vi "Render Draw Line (Clusters).vi"(8 "error in":errorcluster, 9 "End":T1, 10 "Start":T1, 11 "Renderer Pointer":u32 format="%.0x") -> (0 "error out":errorcluster, 3 "Return":i32)   [LabVIEW 2015, in "LibSDL2.lvlib"]
uses:
  LibSDL2.lvlib
  SDL2 Utility/Point (I32).ctl
  DLL/SDL2.dll
  SDL2 Utility/SDL2 Utility.lvlib
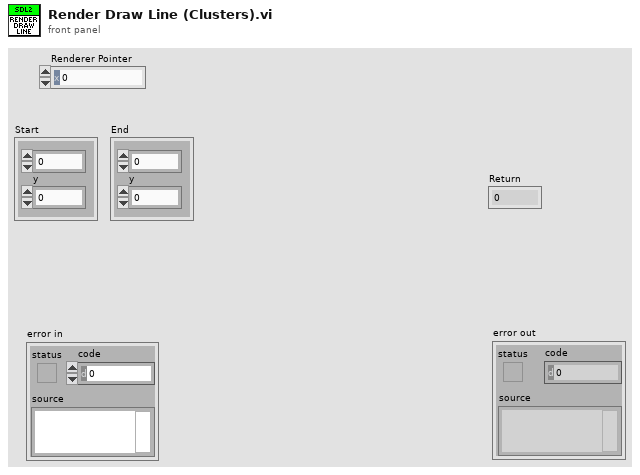
[diagram p1: front panel]
types:
  T1 = typedef "SDL2 Utility.lvlib/Point (I32).ctl" = cluster{"x":i32, "y":i32}
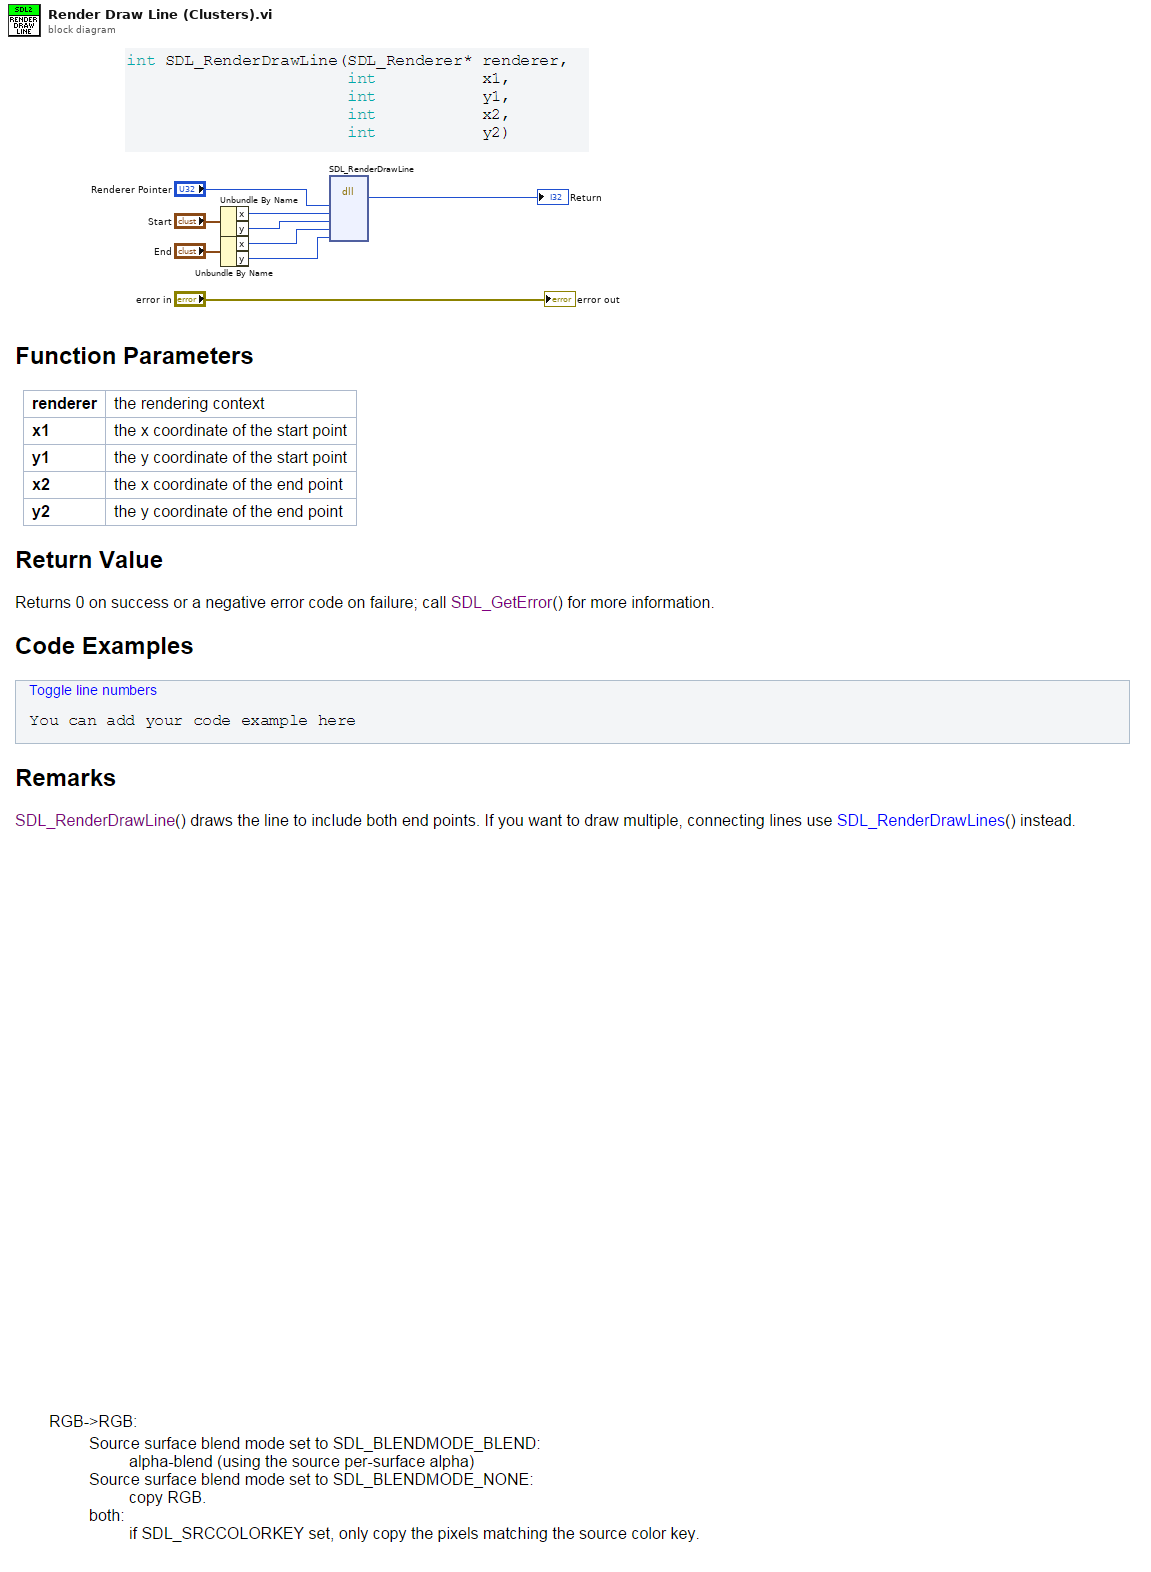
[diagram p0: block diagram]
diagram:
  n1 = Unbundle By Name("Start") -> ("x"=w5:i32, "y"=w4:i32)
  n2 = Unbundle By Name("End") -> ("x"=w2:i32, "y"=w1:i32)
  n3 = dll-call lib="C:/dev/PGS/LabSDL2/Source/Libraries/LibSDL2 Wrapper/DLL/SDL2.dll" fn="SDL_RenderDrawLine"("renderer_pointer"="Renderer Pointer", "x1"=w5, "y1"=w4, "x2"=w2, "y2"=w1) -> ("return type"=→"Return":i32)  [unwired: 8 in, 2 out]
  "error out" <- "error in"
